vi "Ejercicio_01_senal_seno_con_ruido.vi"() -> ()   [LabVIEW 2020]
uses:
  <vilib>/Waveform/WDTOps.llb/WDT Append Waveforms DBL.vi
  <vilib>/measure/maspectr.llb/FFT Power Spectrum and PSD for 1 Chan.vi
  <vilib>/measure/NI_MABase.lvlib
  <vilib>/measure/NI_MAPro.lvlib
panel:
  in  "averaging parameters":T1={"averaging mode"=enum."No averaging", "weighting mode"=enum."Exponential", "number of averages"=10} {"number of averages" min=1}
  in  "stop":bool
  out "Waveform Graph 2":waveform(dbl)(graph)
  out "Waveform Graph":cluster{"f0":dbl, "df":dbl, "magnitude":dbl[]}(graph)
  in  "sampling info":cluster{"Fs":dbl, "#s":dbl}={"Fs"=1000.0, "#s"=1000.0} {"Fs" format="%.2p"}
  in  "Frecuencia":dbl(slide) scale=0.0..500.0
  in  "Amplitud de ruido":dbl(slide) scale=0.0..10.0
  in  "Amplitud":dbl(slide) scale=0.0..10.0
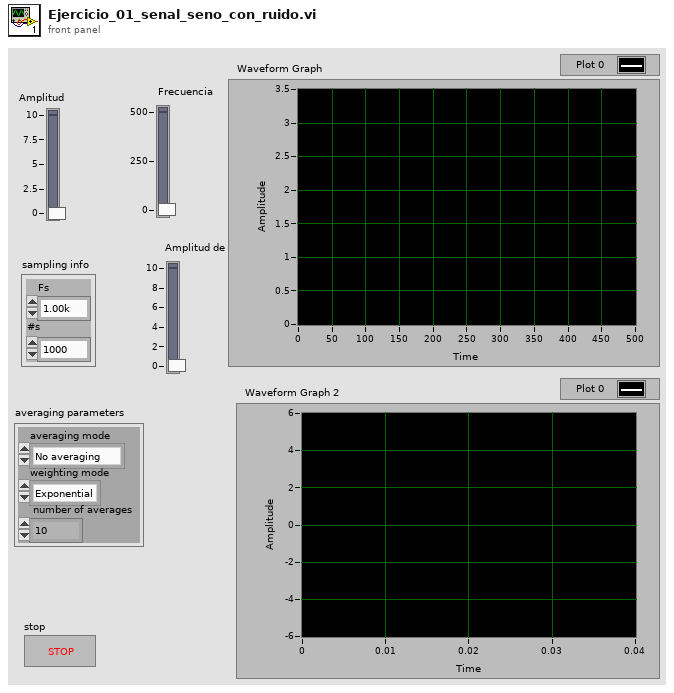
[diagram p1: front panel]
types:
  T1 = cluster{"averaging mode":enum16{"No averaging", "Vector averaging", "RMS averaging", "Peak hold"}, "weighting mode":enum16{"Linear", "Exponential"}, "number of averages":u32}
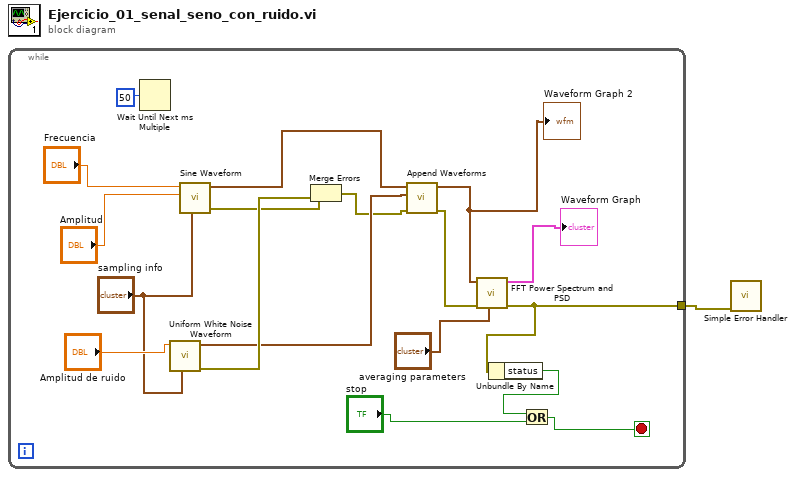
[diagram p0: block diagram]
diagram:
  n1 = while {
    tunnel: [w4] -> w1
    stop <- w5 stop-if-true
    n2 = Wait Until Next ms Multiple(millisecond multiple=u32 50) -> ()  [unwired: 1 out]
    n3 = call <vilib>:"Uniform White Noise Waveform.vi"("sampling info"="sampling info", "amplitude"="Amplitud de ruido") -> ("error out"=w14:errorcluster, "signal out"=w11:waveform(dbl))  [unwired: 8 in]
    n4 = call <vilib>:"Sine Waveform.vi"("sampling info"="sampling info", "amplitude"="Amplitud", "frequency"="Frecuencia") -> ("error out"=w13:errorcluster, "signal out"=w12:waveform(dbl))  [unwired: 7 in]
    n5 = Merge Errors "Merge Errors"(w13, w14) -> (w10:errorcluster)
    n6 = call-poly <vilib>:"Append Waveforms.vi"("error in (no error)"=w10, "waveform B"=w11, "waveform A"=w12) -> ("error out"=w9:errorcluster, "waveform out"=w7:waveform(dbl))  [unwired: 7 in]
    "Waveform Graph 2" <- w7
    n7 = call-poly <vilib>:"FFT Power Spectrum and PSD.vi"("averaging parameters"="averaging parameters", "error in (no error)"=w9, "time signal"=w7) -> ("error out"=w4:errorcluster, "Power Spectrum / PSD"=→"Waveform Graph":cluster{"f0":dbl, "df":dbl, "magnitude":dbl[]})  [unwired: 5 in, 2 out]
    n8 = Unbundle By Name "Unbundle By Name"(w4) -> ("status"=w3:bool)
    n9 = Or(x=w3, y="stop") -> (x .or. y?=w5:bool)
  }
  n10 = call <vilib>:"Simple Error Handler.vi"("error in (no error)"=w1) -> ()  [unwired: 4 in, 5 out]
